vi "ms Time.vi"(1 "error in (no error)":errorcluster) -> (15 "error out":errorcluster, 18 "millisecond timer value":u32)   [LabVIEW 2011]
doc: "Insert a delay with error pass-through to provide data-flow control.\n\n\nVersion 1.0 - 10/21/2009\n\nPhaeron, Inc.\nwww.phaeron.com\ninfo@phaeron.com"
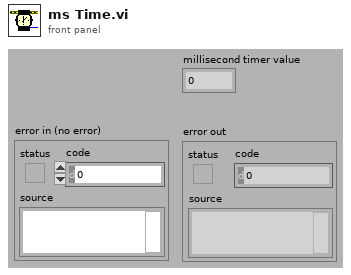
[diagram p1: front panel]
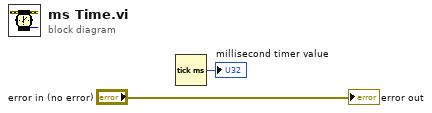
[diagram p0: block diagram]
diagram:
  n1 = Tick Count (ms)() -> (millisecond timer value=→"millisecond timer value":u32)
  "error out" <- "error in (no error)"
